vi "Object detection test.vi"() -> ()   [LabVIEW 2018]
uses:
  Underlying VI's/Modified webcam FGV/Webcam AE.ctl
  <vilib>/userdefined/High Color/IMAQdx.ctl
  Underlying VI's/IMAQ Create Reference AE/IMAQ Reference AE.ctl
panel:
  in  "stop":bool
  out "Image":T1(plugin-control)
  out "Object detection cluster":T2
  out "Object Center Coordinates":cluster{"x":sgl, "y":sgl}
  out "Error out":errorcluster
  in  "Mode":enum16{"Ball", "Soap", "Gel", "Pipe", "None"}(ring)
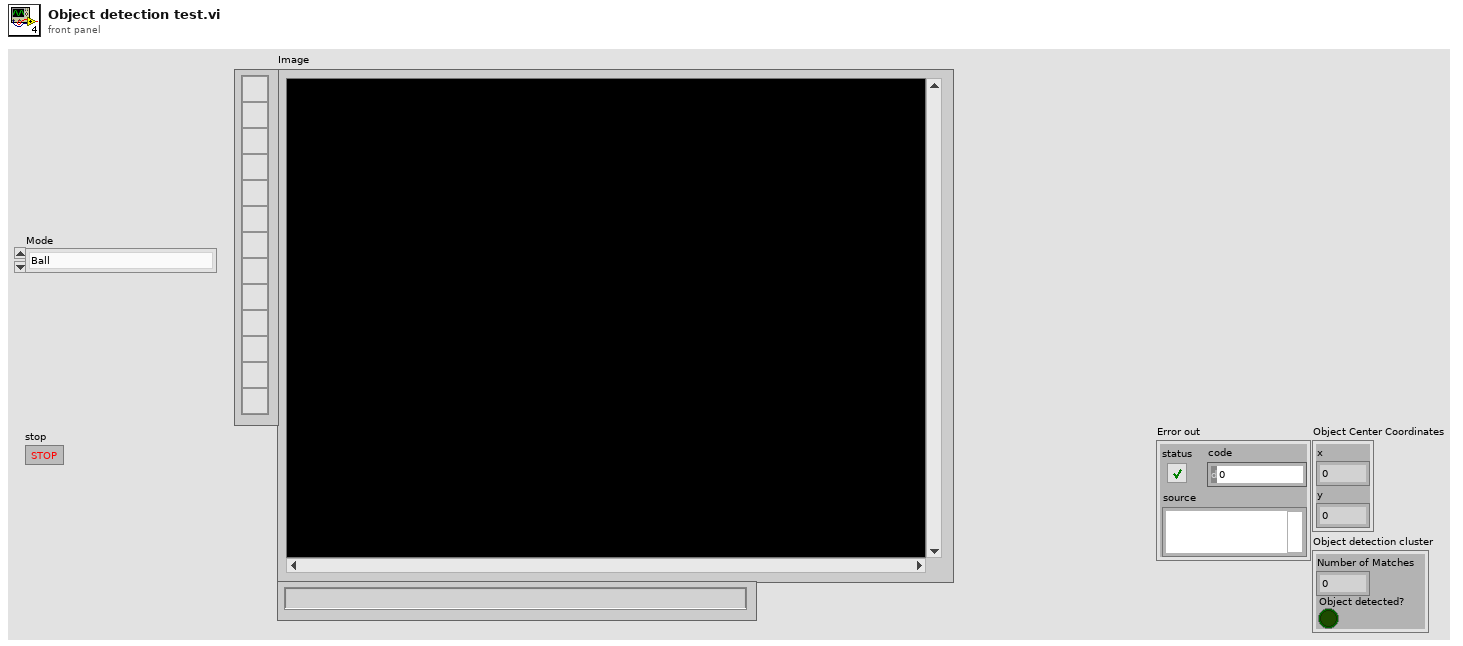
[diagram p1: front panel]
types:
  T1 = typedef "IMAQ Image.ctl" = refnum<image>
  T2 = cluster{"Number of Matches":i32, "Object detected?":bool}
  T3 = typedef "IMAQ Reference AE.ctl" = enum16{"Initialize AE", "Get IMAQ Reference", "Dispose Processing Buffer"}
  T4 = typedef "Webcam AE.ctl" = enum16{"Initialize Camera", "Open Camera", "Continuous Acquisition", "Close Camera", "Retrieve Image", "Dispose Camera Image Buffer"}
  T5 = typedef "IMAQdx.ctl" = refnum<k21>
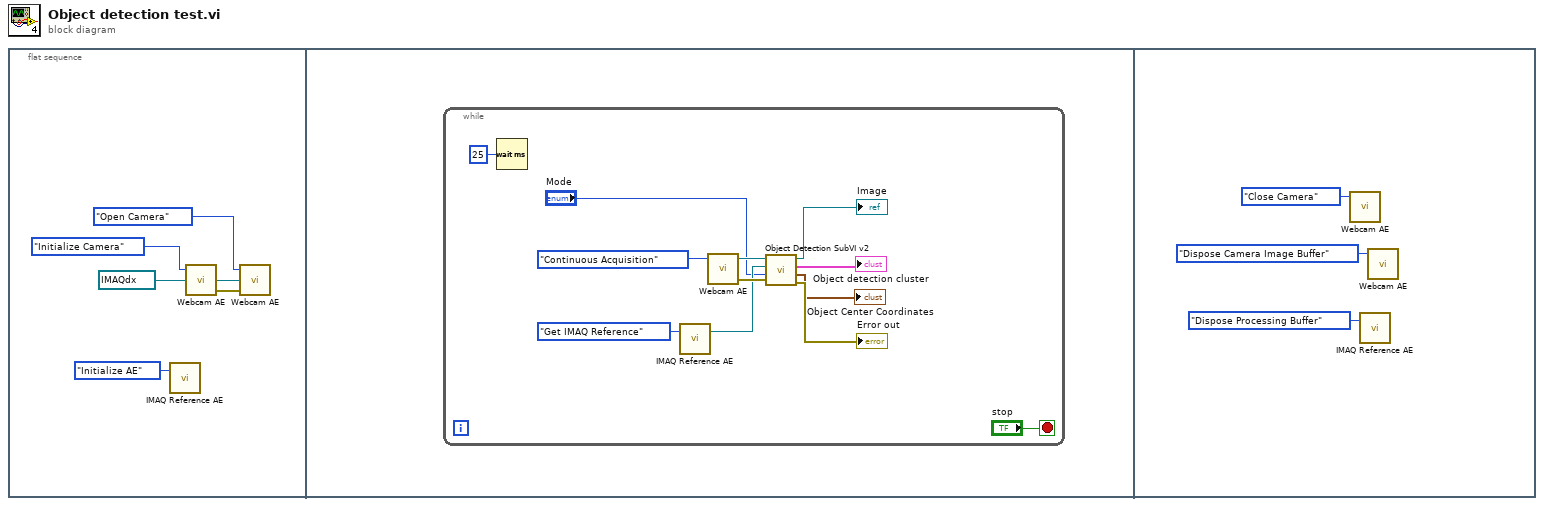
[diagram p0: block diagram]
diagram:
  n1 = flat-sequence {
    frame #0 {
      n2 = call "IMAQ Reference AE.vi"("IMAQ AE States"=IMAQ_Reference_AE."Initialize AE") -> ()  [unwired: 1 in, 2 out]
      n3 = call "Webcam AE.vi"("Session In"=T5 "cam0", "Camera states"=Webcam_AE."Initialize Camera") -> ("error out"=w5:errorcluster, "Session Out"=w6:T5)  [unwired: 1 in, 1 out]
      n4 = call "Webcam AE.vi"("error in (no error)"=w5, "Session In"=w6, "Camera states"=Webcam_AE."Open Camera") -> ()  [unwired: 3 out]
    }
    frame #1 {
      n5 = while {
        stop <- "stop" stop-if-true
        n6 = Wait (ms)(milliseconds to wait=u32 25) -> ()  [unwired: 1 out]
        n7 = call "IMAQ Reference AE.vi"("IMAQ AE States"=IMAQ_Reference_AE."Get IMAQ Reference") -> ("Image Out"=w14:T1)  [unwired: 1 in, 1 out]
        n8 = call "Webcam AE.vi"("Camera states"=Webcam_AE."Continuous Acquisition") -> ("error out"=w18:errorcluster, "Image Out"=w17:T1)  [unwired: 2 in, 1 out]
        n9 = call "Object Detection SubVI v2.vi"("Error In"=w18, "Mode"="Mode", "Image Dest"=w14, "Image in"=w17) -> ("Error out"=→"Error out":errorcluster, "Object Center Coordinates"=→"Object Center Coordinates":cluster{"x":sgl, "y":sgl}, "Object detection cluster"=→"Object detection cluster":T2, "Image Out"=→"Image":T1)
      }
    }
    frame #2 {
      n10 = call "Webcam AE.vi"("Camera states"=Webcam_AE."Close Camera") -> ()  [unwired: 2 in, 3 out]
      n11 = call "IMAQ Reference AE.vi"("IMAQ AE States"=IMAQ_Reference_AE."Dispose Processing Buffer") -> ()  [unwired: 1 in, 2 out]
      n12 = call "Webcam AE.vi"("Camera states"=Webcam_AE."Dispose Camera Image Buffer") -> ()  [unwired: 2 in, 3 out]
    }
  }
